vi "Read_Data_All.vi"(7 "gain":dbl format="%#_6f", 10 "samples per read":i32, 11 "path":path) -> (0 "error out":errorcluster, 1 "runtime (ms)":dbl format="%#_6f", 3 "Complex Out":cdb[][](array[numeric]))   [LabVIEW 2016]
uses:
  <instrlib>/niRFSG/niRFSG.llb/niRFSG Write Arb Waveform (I-Q).vi
panel:
  out "element":i16
  out "Waveform Graph":dbl[](graph)
  out "Samples Written":dbl format="%#.6g"
  in  "element 3":string
  in  "Direct Download":i32(ring)=1 items=["Disable", "Enable"]
  in  "Pre-filter Gain (dB)":dbl=-2.0 format="%_3f"
  in  "Power Level [dBm]":dbl=-20.0 format="%_3f"
  in  "Number of Samples Per Write":i32=64000 format="%#.6g"
  in  "IQ Rate (S/s)":dbl=8333333.0 format="%#.3p"
  in  "Signal Bandwidth":dbl=5000000.0 format="%#.3p"
  in  "Center Frequency [Hz]":dbl=1000000000.0 format="%#.3p"
  in  "Power Level Type":i32(ring)=7001 items=["Average Power"=7000, "Peak Power"=7001]
  out "Total Number Of Samples":dbl format="%#.6g"
  out "Actual IQ Rate (S/s)":dbl=8333333.333333333 format="%#.3p"
  out "Generating":bool
  in  "Stop":bool
  in  "Tab Control":enum32{"Page 1", "Page 2"}(tab)
  out "Progress Bar":dbl(slide) scale=0.0..100.0
  out "file size (in samples)":dbl format="%#_6f"
  out "start time (ms)":u32
  out "stop time (ms)":u32
  in  "byte order":T1(ring)
  out "cancelled":bool
  # "Setup Input"
  # "Runtime Output"
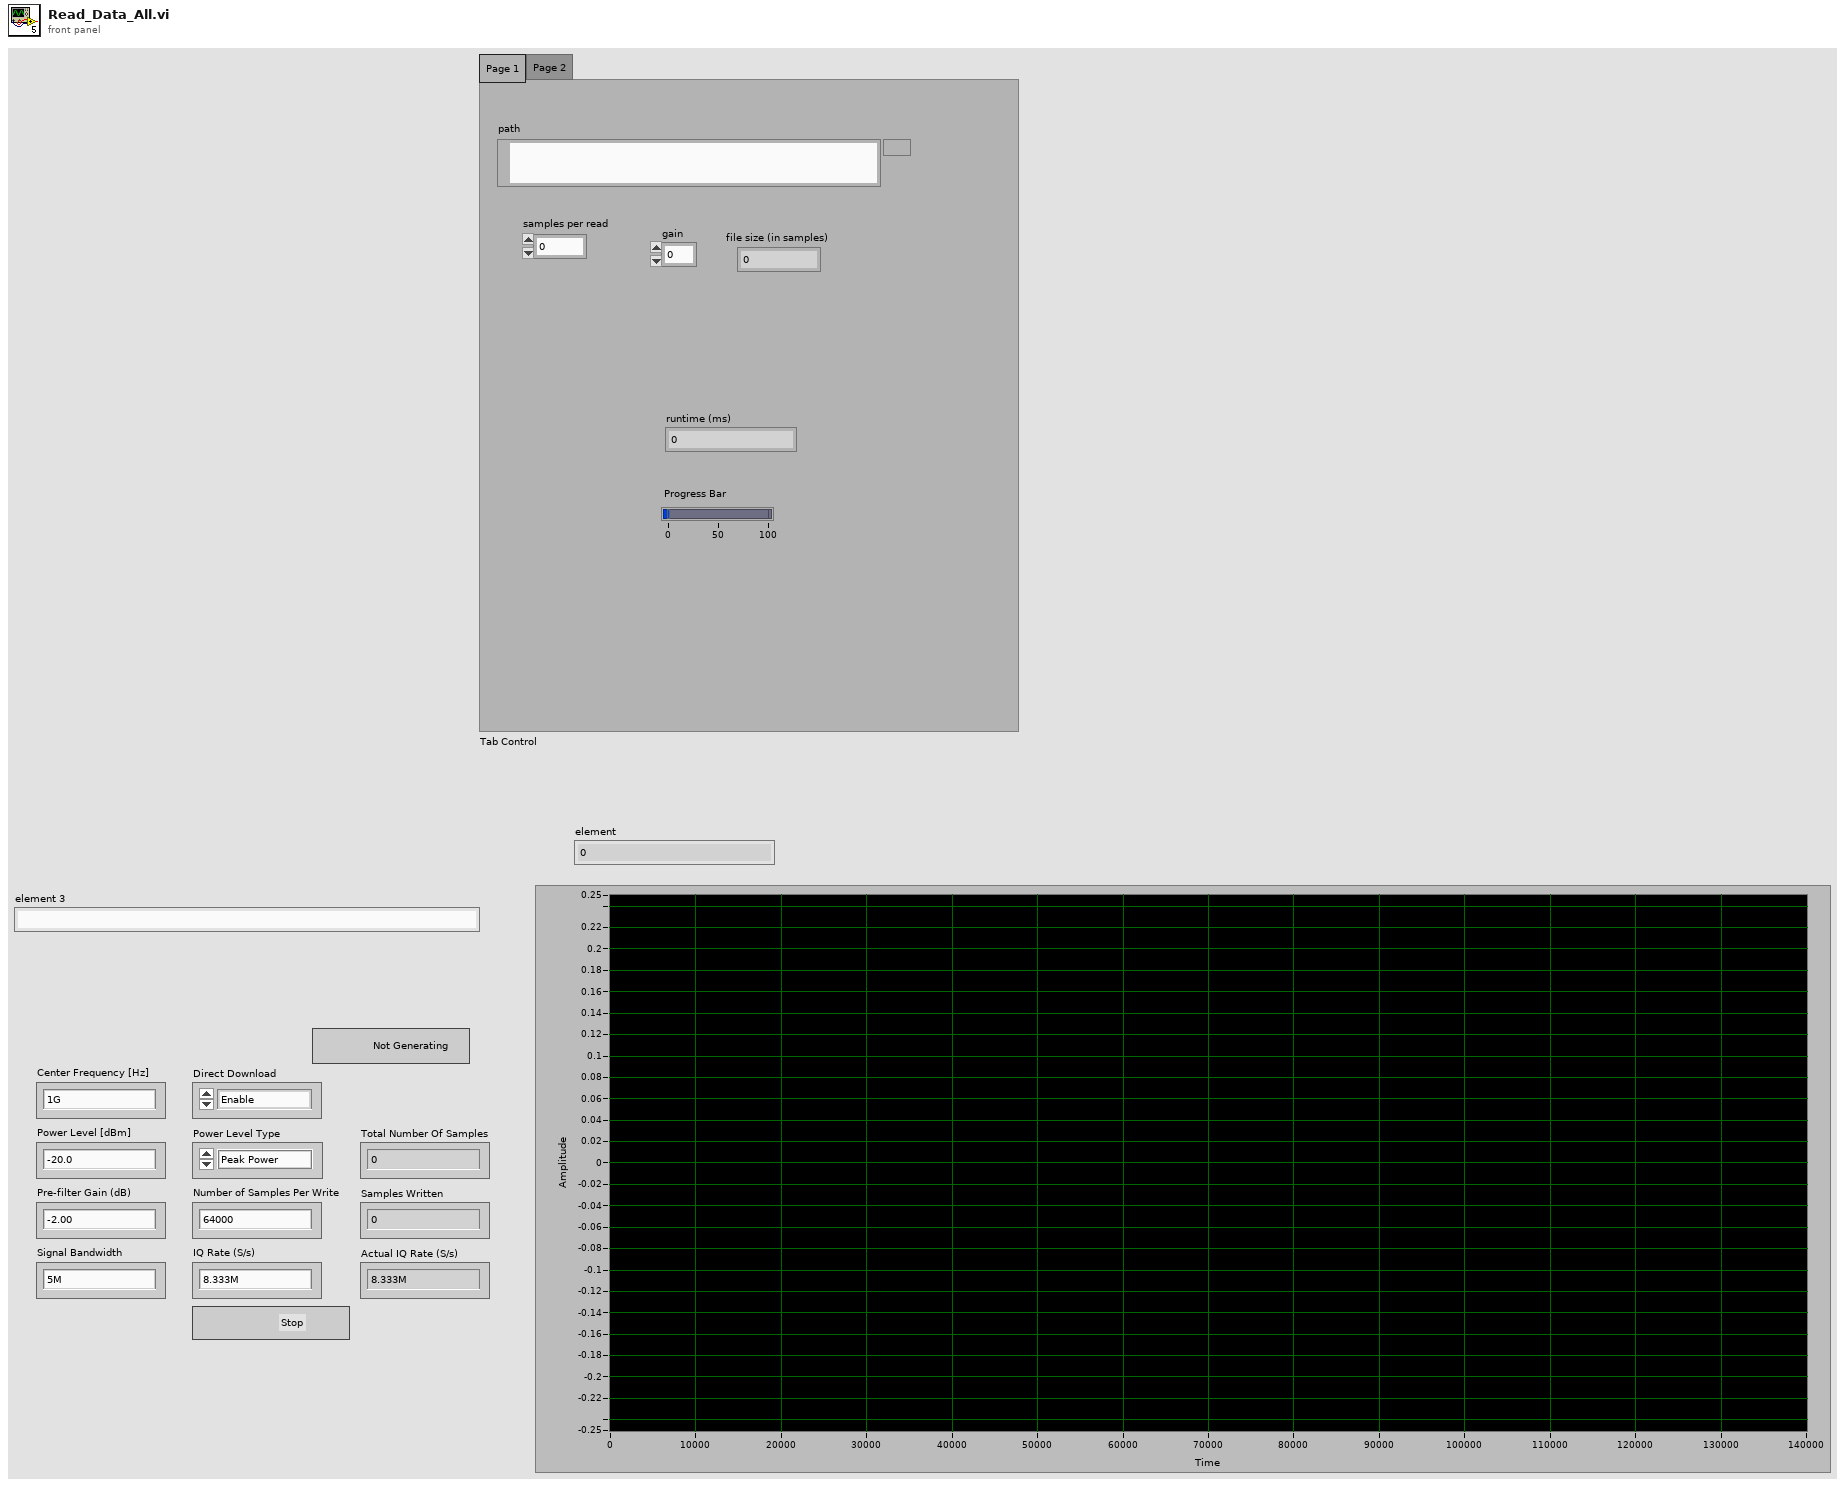
[diagram p1: front panel]
types:
  T1 = enum16{"big-endian, network order", "native, host order", "little-endian"}
  T2 = enum16{"open", "replace", "create", "open or create", "replace or create", "replace or create with confirmation"}
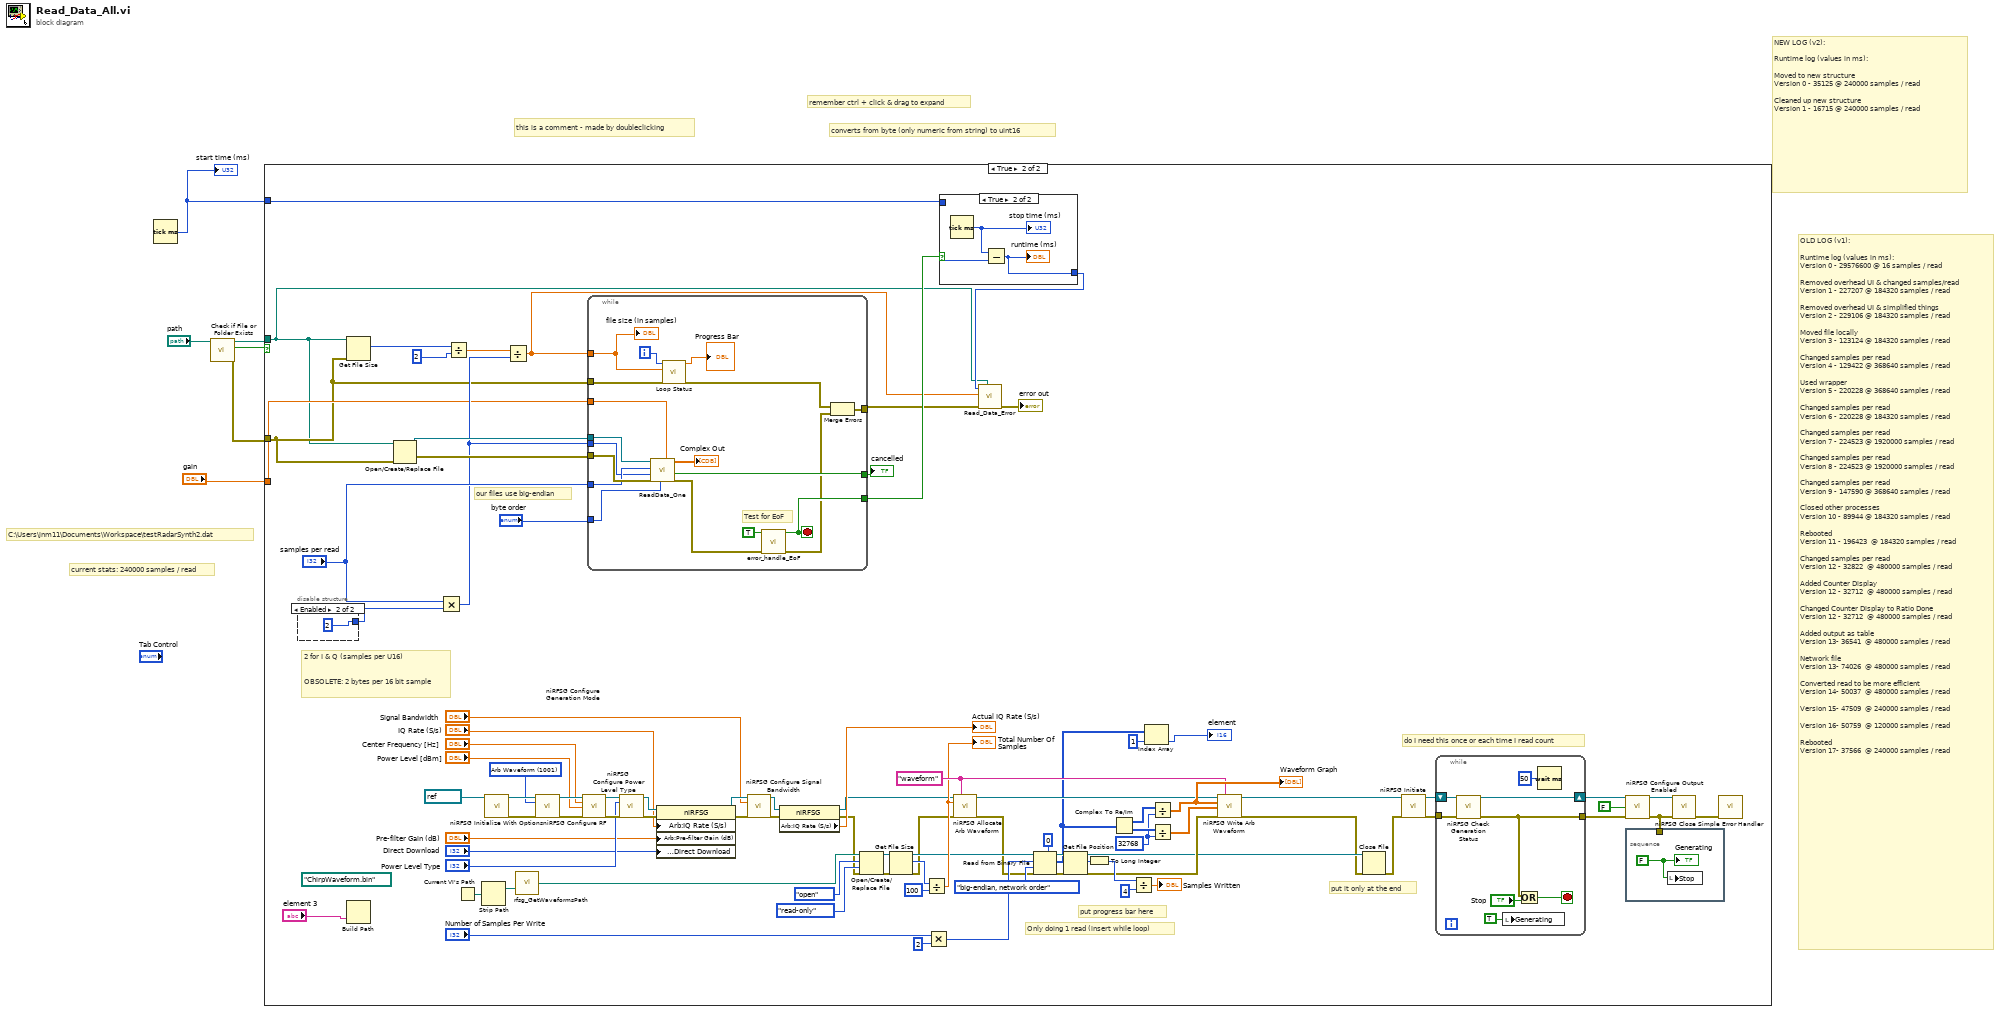
[diagram p0: block diagram]
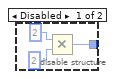
[diagram p3: hidden frame]
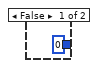
[diagram p4: hidden frame]
diagram:
  # "NEW LOG (v2):\n\nRuntime log (values in ms):\n\nMoved to new structure\nVersion 0 - 35125 @ 240000 samples / read\n\nCleaned up new structure\nVersion 1 - 16715 @ 240000 samples / read"
  # "current stats: 240000 samples / read"
  # "C:\\Users\\jnm11\\Documents\\Workspace\\testRadarSynth2.dat"
  # "OLD LOG (v1):\n\nRuntime log (values in ms):\nVersion 0 - 29576600 @ 16 samples / read\n\nRemoved overhead UI & changed samples/read\nVersion 1 - 227207 @ 184320 samples / read\n\nRemoved overhead UI & simplified things \nVersion 2 - 229106 @ 184320 samples / read\n\nMoved file locally\nVersion 3 - 123124 @ 184320 samples / read\n\nChanged samples per read\nVersion 4 - 129422 @ 368640 samples / read\n\nUsed wrapper\nVersion 5 - 220228 @ 368640 samples / read\n\nChanged samples per read\nVersion 6 - 220228 @ 184320 samples / read\n\nChanged samples per read\nVersion 7 - 224523 @ 1920000 samples / read\n\nChanged samples per read\nVersion 8 - 224523 @ 1920000 samples / read\n\nChanged samples per read\nVersion 9 - 147590 @ 368640 samples / read\n\nClosed other processes\nVersion 10 - 89944 @ 184320 samples / read\n\nRebooted\nVersion 11 - 196423  @ 184320 samples / read\n\nChanged samples per read\nVersion 12 - 32822  @ 480000 samples / read\n\nAdded Counter Display\nVersion 12 - 32712  @ 480000 samples / read\n\nChanged Counter Display to Ratio Done\nVersion 12 - 32712  @ 480000 samples / read\n\nAdded output as table\nVersion 13- 36541  @ 480000 samples / read\n\nNetwork file\nVersion 13- 74026  @ 480000 samples / read\n\nConverted read to be more efficient\nVersion 14- 50037  @ 480000 samples / read\n\nVersion 15- 47509  @ 240000 samples / read\n\nVersion 16- 50759  @ 120000 samples / read\n\nRebooted\nVersion 17- 37566  @ 240000 samples / read"
  # "converts from byte (only numeric from string) to uint16"
  # "remember ctrl + click & drag to expand"
  # "this is a comment - made by doubleclicking"
  n1 = Tick Count (ms)() -> (millisecond timer value=w2:u32)
  "start time (ms)" <- w2
  n2 = call <vilib>:"Check if File or Folder Exists.vi"("path"="path") -> ("error out"=w3:errorcluster, "file or folder exists?"=w4:bool, "dup path"=w5:path)  [unwired: 8 in]
  n3 = case shown="True" w4 {
    tunnel: w5 -> [_ w80]
    tunnel: w3 -> [_ w85]
    tunnel: w2 -> [_ w94]
    tunnel: "gain" -> [_ w86]
    frame False {
    }
    frame True {
      w65 = path "ChirpWaveform.bin" ("Waveform File Path (dialog if empty)")
      w66 = 32768
      w58 = 1001 items=["CW"=1000, "Arb Waveform"=1001, "Script"=1002] ("generation mode")
      w57 = "waveform" ("name")
      # "do I need this once or each time I read count"
      # "put it only at the end"
      # "put progress bar here"
      # "Only doing 1 read (insert while loop)"
      # "2 for I & Q (samples per U16)\n\n\nOBSOLETE: 2 bytes per 16 bit sample"
      # "our files use big-endian"
      n4 = disable-structure shown="Enabled" {
        disable-tunnel: [w108 2 ("y")] -> w92
        frame Disabled {
          n5 = Multiply(x=2 ("column N"), y=2 ("column N")) -> (x*y=w108:i32)
        }
        frame Enabled {
        }
      }
      n6 = Get File Size(file=w80, error in=w85) -> (size (in bytes)=w91:i64)  [unwired: 2 out]
      n7 = Build Path(name or relative path="element 3") -> ()  [unwired: 1 in, 1 out]
      n8 = Open/Create/Replace File(file path (use dialog)=w80, error in=w85) -> (refnum out=w98:refnum<file>, error out=w97:errorcluster)  [unwired: 4 in, 1 out]
      n9 = Multiply(x="samples per read", y=w92) -> (x*y=w88:i32)
      n10 = Divide(x=w91, y=i64 2) -> (x/y=w89:dbl)
      n11 = Current VI's Path() -> (path=w42:path)
      n12 = Strip Path(path=w42) -> (stripped path=w43:path)  [unwired: 1 out]
      n13 = call <instrlib>:"niRFSG Initialize With Options.vi"("resource name"=refnum<k15> "VST" ("Resource Name")) -> ("instrument handle"=w62:refnum<k15>, "error out"=w63:errorcluster)  [unwired: 13 in]
      n14 = Divide(x=w89, y=w88) -> (x/y=w82:dbl)
      n15 = call <instrlib>:"rfsg_GetWaveformsPath.vi"("path relative to"=w43) -> ("waveforms path"=w34:path)  [unwired: 14 in]
      n16 = call <instrlib>:"niRFSG Configure Generation Mode.vi"("instrument handle"=w62, "generation mode"=w58, "error in"=w63) -> ("instrument handle out"=w50:refnum<k15>, "error out"=w49:errorcluster)  [unwired: 11 in]
      n17 = call <instrlib>:"niRFSG Configure RF.vi"("instrument handle"=w50, "frequency (Hz)"="Center Frequency [Hz]", "power level (dBm)"="Power Level [dBm]", "error in"=w49) -> ("instrument handle out"=w40:refnum<k15>, "error out"=w38:errorcluster)  [unwired: 10 in]
      n18 = while {
        tunnel: w98 -> [w127]
        tunnel: w97 -> [w131]
        tunnel: "byte order" -> [w128]
        tunnel: w88 -> [w129]
        tunnel: "samples per read" -> [w130]
        tunnel: w82 -> [w123]
        tunnel: [w126] -> w93
        tunnel: [w132] -> w87
        tunnel: [w116] -> w84
        tunnel: w86 -> [w119]
        tunnel: w85 -> [w121]
        i -> [w122]
        stop <- w126 stop-if-true
        # "Test for EoF"
        n19 = call "ReadData_One"("gain"=w119, "byte order (0:big-endian, network order)"=w128, "error in"=w131, "words per read (uint16)"=w129, "samples per read"=w130, "file refnum"=w127) -> ("error out"=w124:errorcluster, "cancelled"=w132:bool, "Complex Out"=→"Complex Out":cdb[][])  [unwired: 3 in]
        n20 = call "Loop Status.vi"("error in"=w121, "total count"=w123, "current count"=w122) -> ("error out"=w117:errorcluster, "total count"=→"Progress Bar":dbl)  [unwired: 7 in]
        n21 = call "error_handle_EoF.vi"("error in"=w124, "Remove EoF Error?"=TRUE ("NON-FUNCTIONAL: Remove EoF Error?")) -> ("error out"=w118:errorcluster, "is EoF?"=w126:bool)  [unwired: 7 in, 1 out]
        n22 = Merge Errors(w117, w118) -> (w116:errorcluster)
        "file size (in samples)" <- w123
      }
      "cancelled" <- w87
      n23 = call <instrlib>:"niRFSG Configure Power Level Type.vi"("instrument handle"=w40, "power level type"="Power Level Type", "error in"=w38) -> ("instrument handle out"=w39:refnum<k15>, "error out"=w37:errorcluster)  [unwired: 11 in]
      n24 = property on="Property Node" class="niRFSG"(reference=w39, error in=w37, "Arb:IQ Rate (S/s)"="IQ Rate (S/s)", "Arb:Pre-filter Gain (dB)"="Pre-filter Gain (dB)", "Arb:Data Transfer:Direct Download"="Direct Download") -> (reference out=w41:refnum<k15>, error out=w28:errorcluster)
      n25 = call <instrlib>:"niRFSG Configure Signal Bandwidth.vi"("instrument handle"=w41, "signal bandwidth (Hz)"="Signal Bandwidth", "error in"=w28) -> ("instrument handle out"=w27:refnum<k15>, "error out"=w25:errorcluster)  [unwired: 11 in]
      n26 = property class="niRFSG"(reference=w27, error in=w25) -> (reference out=w26:refnum<k15>, error out=w24:errorcluster, "Arb:IQ Rate (S/s)"=→"Actual IQ Rate (S/s)":dbl)
      n27 = Open/Create/Replace File(file path (use dialog)=w34, error in=w24, operation (0:open)=T2."open", access (0:read/write)=enum16{"read/write", "read-only", "write-only"}."read-only") -> (refnum out=w31:refnum<file>, error out=w33:errorcluster)  [unwired: 2 in, 1 out]
      n28 = Get File Size(file=w31, error in=w33) -> (refnum out=w30:refnum<file>, size (in bytes)=w32:i64, 0:w23:errorcluster)
      n29 = Divide(x=w32, y=100) -> (x/y=w46:dbl)
      "Total Number Of Samples" <- w46
      n30 = Multiply(x="Number of Samples Per Write", y=2) -> (x*y=w44:i32)
      n31 = case shown="True" w93 {
        tunnel: w94 -> [_ w114]
        tunnel: [u32 0 w113] -> w81
        frame False {
        }
        frame True {
          n32 = Tick Count (ms)() -> (millisecond timer value=w115:u32)
          "stop time (ms)" <- w115
          n33 = Subtract(x=w115, y=w114) -> (x-y=w113:u32)
          "runtime (ms)" <- w113
        }
      }
      n34 = call <instrlib>:"niRFSG Allocate Arb Waveform.vi"("instrument handle"=w26, "name"=w57, "size in samples"=w46, "error in"=w23) -> ("instrument handle out"=w59:refnum<k15>, "error out"=w11:errorcluster)  [unwired: 10 in]
      n35 = call "Read_Data_Error.vi"("path"=w80, "error in (no error)"=w84, "file size (in samples)"=w82, "runtime"=w81) -> ("error out"=→"error out":errorcluster)  [unwired: 7 in]
      n36 = Read from Binary File(5:i16 0 ("I16"), 8:w11, 9:T1."big-endian, network order" ("byte order (0:big-endian, network order)"), 10:w44, 11:w30) -> (0:w75:errorcluster, 2:w8:i16[], 3:w74:refnum<file>)  [unwired: 1 in, 1 out]
      n37 = Get File Position(4:w75, 7:w74) -> (0:w67:errorcluster, 2:w76:i64, 3:w48:refnum<file>)
      n38 = To Long Integer(number=w76) -> (32bit integer=w71:i32)
      n39 = Complex To Re/Im(x + iy=w8) -> (x=w68:i16[], y=w69:i16[])
      n40 = Divide(x=w71, y=4) -> (x/y=→"Samples Written":dbl)
      n41 = Index Array(array=w8, index=1) -> (element=→"element":i16)
      n42 = Divide(x=w68, y=w66) -> (x/y=w79:dbl[])
      "Waveform Graph" <- w79
      n43 = Divide(x=w69, y=w66) -> (x/y=w78:dbl[])
      n44 = call-poly <instrlib>:"niRFSG Write Arb Waveform.vi"("instrument handle"=w59, "name"=w57, "I Data"=w79, "Q Data"=w78, "error in"=w67) -> ("instrument handle out"=w56:refnum<k15>, "error out"=w12:errorcluster)  [unwired: 9 in]
      n45 = Close File(refnum=w48, error in=w12) -> (error out=w47:errorcluster)  [unwired: 1 out]
      n46 = call <instrlib>:"niRFSG Initiate.vi"("instrument handle"=w56, "error in"=w47) -> ("instrument handle out"=w55:refnum<k15>, "error out"=w13:errorcluster)  [unwired: 12 in]
      n47 = while {
        shift-right: [w106] -> w54
        shift-left: w55 -> [w107]
        tunnel: [w101] -> w14
        tunnel: w13 -> [w100]
        stop <- w104 stop-if-true
        n48 = call <instrlib>:"niRFSG Check Generation Status.vi"("instrument handle"=w107, "error in"=w100) -> ("instrument handle out"=w106:refnum<k15>, "error out"=w101:errorcluster)  [unwired: 11 in, 1 out]
        n49 = local write "Generating"(TRUE ("Boolean")) -> ()
        n50 = Or(x=w101, y="Stop") -> (x .or. y?=w104:bool)
        n51 = Wait (ms)(milliseconds to wait=u32 50) -> ()  [unwired: 1 out]
      }
      n52 = call <instrlib>:"niRFSG Configure Output Enabled.vi"("instrument handle"=w54, "output enabled"=FALSE ("output enable"), "error in"=w14) -> ("instrument handle out"=w61:refnum<k15>, "error out"=w53:errorcluster)  [unwired: 11 in]
      n53 = stacked-sequence {
        tunnel: w53 -> [_]
        frame #0 {
          w99 = FALSE ("Boolean")
          n54 = local write "Stop"(w99) -> ()
          "Generating" <- w99
        }
      }
      n55 = call <instrlib>:"niRFSG Close.vi"("instrument handle"=w61, "error in"=w53) -> ("error out"=w15:errorcluster)  [unwired: 13 in]
      n56 = call <vilib>:"Simple Error Handler.vi"("error in (no error)"=w15) -> ()  [unwired: 4 in, 5 out]
    }
  }
